vi "oa_Check Spectral Map Settings (Time).vi"(7 "reset in":bool, 8 "error in (no error)":errorcluster, 10 "speed profile":T1 {"speed [RPM]" format="%.2f"; "time [s]" format="%.2f"}, 11 "segment":cluster{"start":dbl, "end":dbl, "step":dbl} {"step" format="%.2f"; "end" format="%.2f"; "start" format="%.2f"}) -> (0 "error out":errorcluster, 2 "speed profile out":T1 {"speed [RPM]" format="%.2f"; "time [s]" format="%.2f"}, 3 "segment out":cluster{"start":dbl, "end":dbl, "step":dbl} {"step" format="%.2f"; "end" format="%.2f"; "start" format="%.2f"}, 4 "step found?":bool, 5 "reset out":bool)   [LabVIEW 2017, in "SoundVib_Resampling.lvlib"]
uses:
  <vilib>/addons/Sound and Vibration/Order Analysis/Resample Order Tracking/SoundVib_Resampling.lvlib
  <vilib>/addons/Sound and Vibration/Order Analysis/Tach Process/SubVIs/speed profile.ctl
  <vilib>/addons/Sound and Vibration/Order Analysis/Tach Process/SoundVib_TachProcess.lvlib
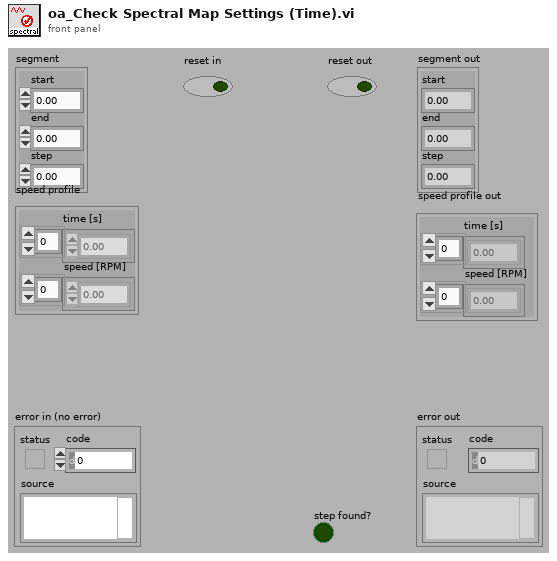
[diagram p1: front panel]
types:
  T1 = typedef "SoundVib_TachProcess.lvlib/speed profile.ctl" = cluster{"time [s]":dbl[], "speed [RPM]":dbl[]}
  T2 = cluster{"start (s)":dbl, "end (s)":dbl, "step (s)":dbl}
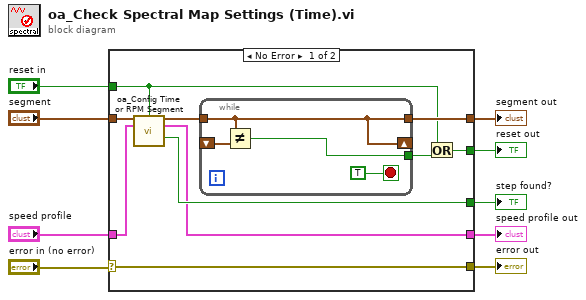
[diagram p0: block diagram]
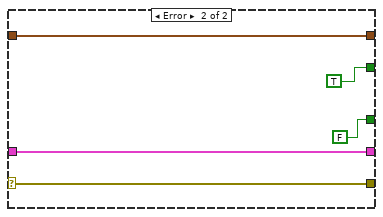
[diagram p2: hidden frame]
diagram:
  n1 = case shown="No Error" "error in (no error)" {
    selector: "error in (no error)" -> [w18 w28]
    tunnel: [w18 w28] -> w8
    tunnel: "segment" -> [w17 w26]
    tunnel: [w13 TRUE] -> w6
    tunnel: [w19 w26] -> w5
    tunnel: "speed profile" -> [w11 w25]
    tunnel: [w10 w25] -> w3
    tunnel: "reset in" -> [w14 _]
    tunnel: [w12 FALSE ("step found?")] -> w1
    frame No Error {
      n2 = call <vilib>:"oa_Config Time or RPM Segment.vi"("time segment"=w17, "reset in"=w14, "speed profile"=w11) -> ("time segment out"=w16:T2, "speed profile out"=w10:T1, "step found?"=w12:bool)  [unwired: 7 in, 3 out]
      n3 = while {
        tunnel: w16 -> [w21]
        shift-right: [w21] -> _
        shift-left: _ -> [w22]
        tunnel: [w20] -> w15
        tunnel: [w21] -> w19
        stop <- TRUE stop-if-true
        n4 = Not Equal?(x=w21, y=w22) -> (x != y?=w20:bool)
      }
      n5 = Or(x=w14, y=w15) -> (x .or. y?=w13:bool)
    }
    frame Error {
    }
  }
  "error out" <- w8
  "segment out" <- w5
  "reset out" <- w6
  "speed profile out" <- w3
  "step found?" <- w1
